vi "get_pdo_node.vi"(10 "node":u8, 11 "index":u16) -> (2 "node":u8, 3 "return":i16)   [LabVIEW 2011]
uses:
  canopen_dll_master.dll
panel:
  in  "node":cluster{"node":u8}
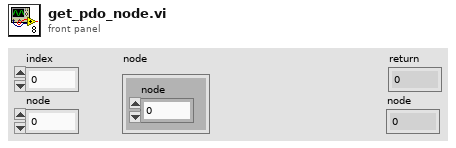
[diagram p1: front panel]
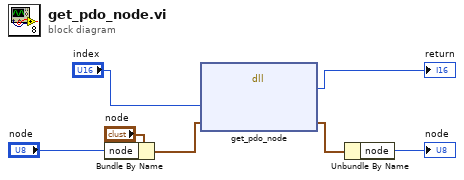
[diagram p0: block diagram]
diagram:
  n1 = Bundle By Name(cluster="node", "node"="node") -> (w4:cluster{"node":u8})
  n2 = dll-call lib="canopen_dll_master.dll" fn="get_pdo_node"("index"="index", "node"=w4) -> ("return type"=→"return":i16, "node"=w1:cluster{"node":u8})  [unwired: 4 in, 2 out]
  n3 = Unbundle By Name(w1) -> ("node"=→"node":u8)
